vi "Wait(ms) with error-clusters.vi"(4 "Error In":errorcluster, 7 "wait (msec)":u32) -> (0 "Error Out":errorcluster)   [LabVIEW 2014, in "Timing.lvlib"]
uses:
  Timing.lvlib
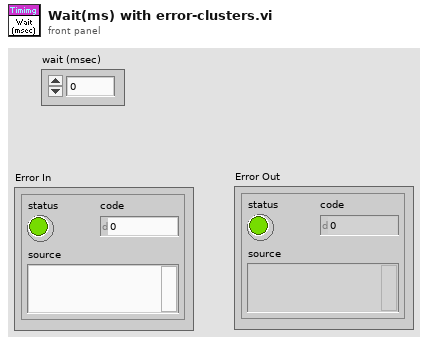
[diagram p1: front panel]
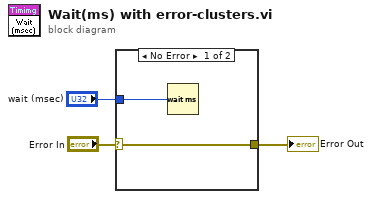
[diagram p0: block diagram]
diagram:
  n1 = case shown="No Error" "Error In" {
    selector: "Error In" -> [w5 w6]
    tunnel: [w5 w6] -> w3
    tunnel: "wait (msec)" -> [w4 _]
    frame No Error {
      n2 = Wait (ms)(milliseconds to wait=w4) -> ()  [unwired: 1 out]
    }
    frame Error {
    }
  }
  "Error Out" <- w3
